vi "A 正面 处理函数.vi"(8 "error in (no error)":errorcluster caption="错误输入（无错误）", 10 "Image Name":string="I1", 11 "ParamsUI":T1 caption="参数界面" {"Exposure Values" scale=0.0..200000.0}) -> (0 "error out":errorcluster caption="错误输出", 3 "Image out":T3(plugin-control))   [LabVIEW 2015]
uses:
  <vilib>/userdefined/High Color/IMAQdx.ctl
  <resource>/objmgr/imaqdx.rc
  <vilib>/vision/driver/NI_Vision_Acquisition_Software.lvlib
panel:
  in  "Session Out":T2
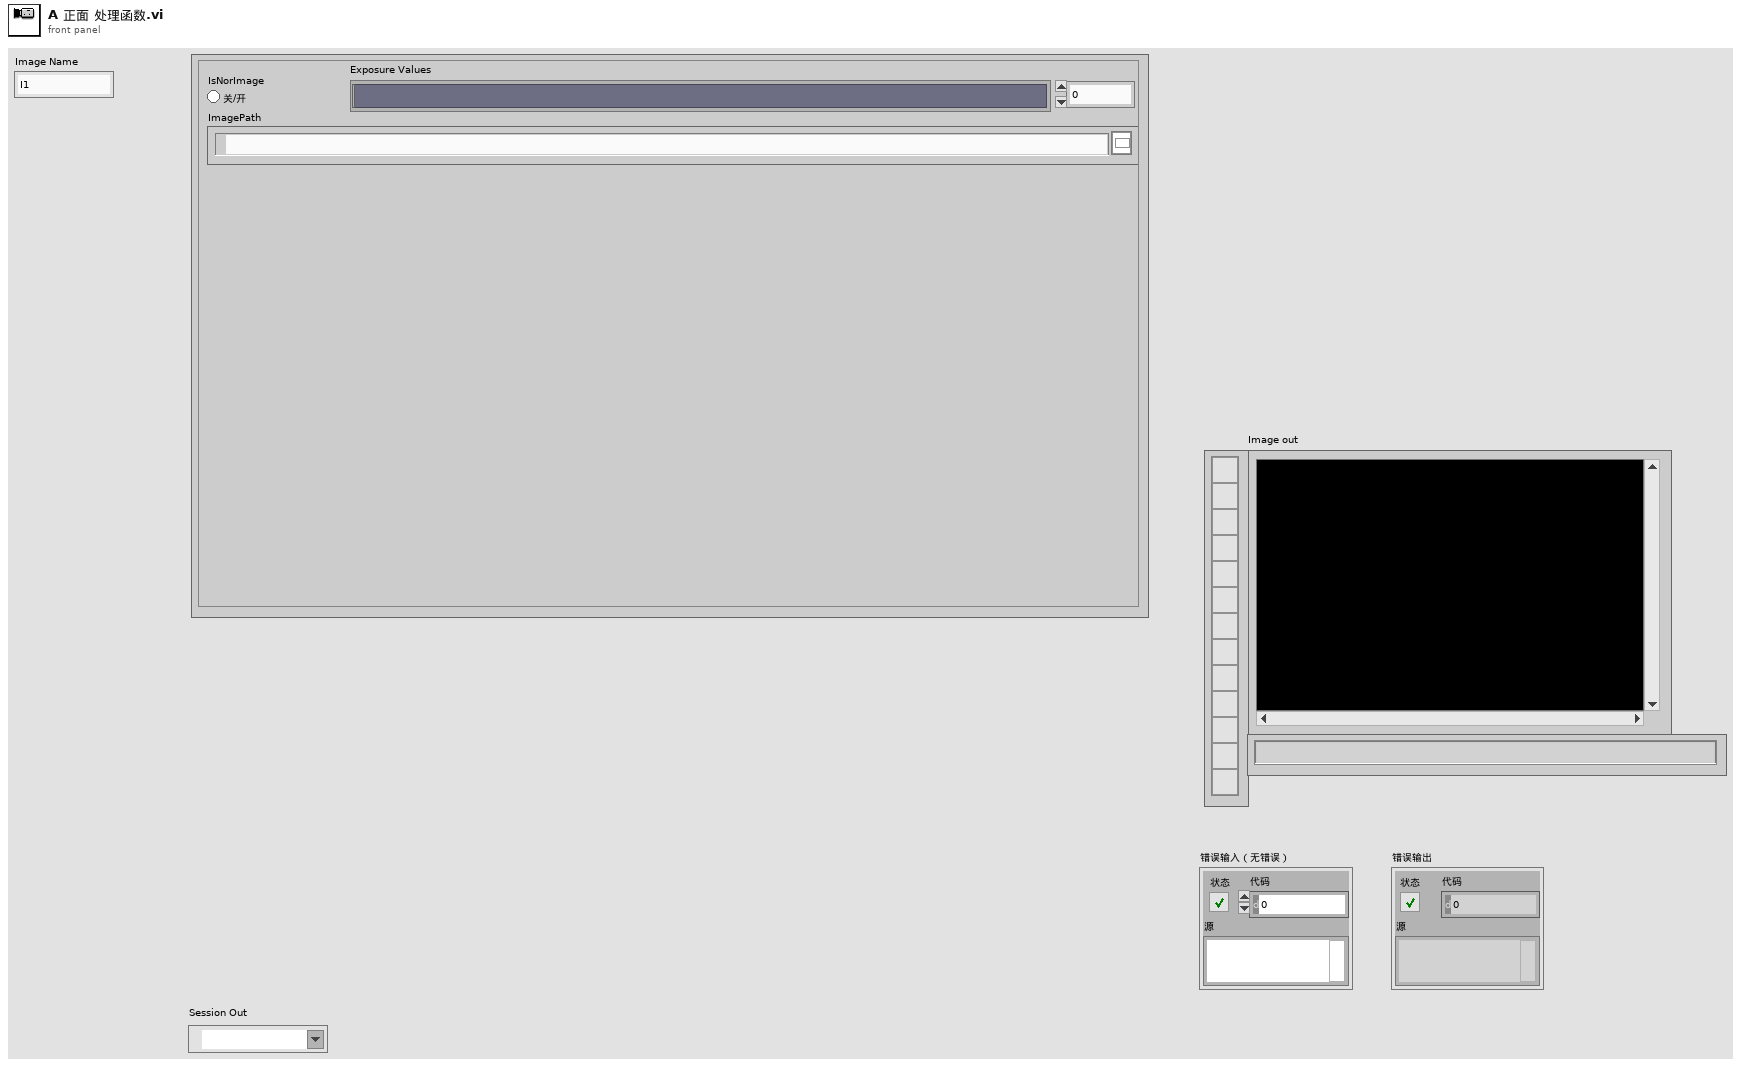
[diagram p1: front panel]
types:
  T1 = cluster{"IsNorImage":bool, "Exposure Values":u32, "ImagePath":path}
  T2 = typedef "IMAQdx.ctl" = refnum<k21>
  T3 = typedef "IMAQ Image.ctl" = refnum<image>
  T4 = typedef "Image Type" = u32
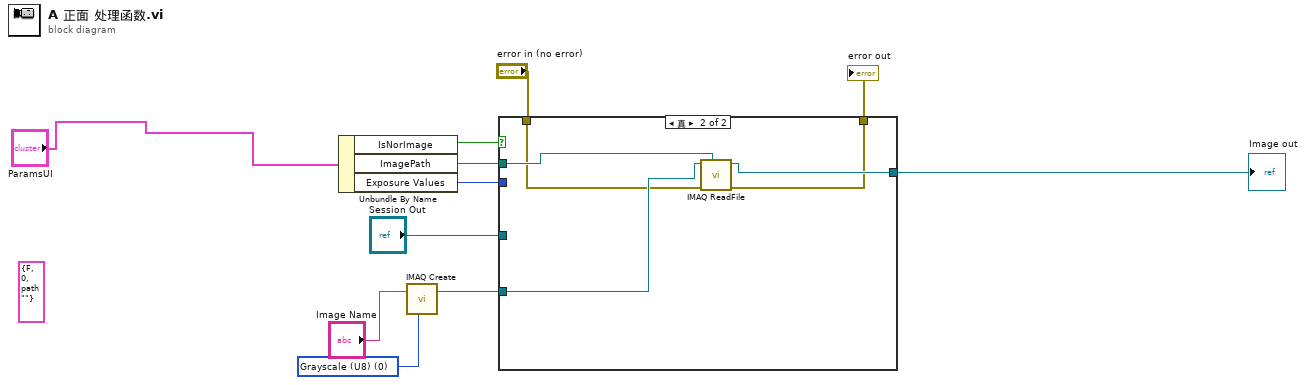
[diagram p0: block diagram]
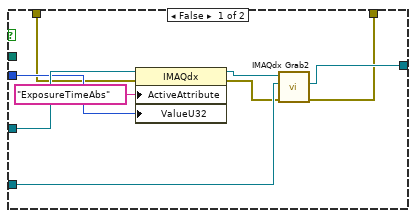
[diagram p2: hidden frame]
diagram:
  w1 = T4 0 items=["Grayscale (U8)", "Grayscale (I16)", "Grayscale (SGL)", "Complex (CSG)", "RGB (U32)", "HSL (U32)", "RGB (U64)", "Grayscale (U16)"] ("Image Type")
  (unwired) T1 {"IsNorImage"=FALSE, "Exposure Values"=0, "ImagePath"=path ""} ("ParamsUI")
  n1 = Unbundle By Name("ParamsUI") -> ("IsNorImage"=w11:bool, "ImagePath"=w10:path, "Exposure Values"=w8:u32)
  n2 = call "IMAQ Create"("Image Name"="Image Name", "Image Type"=w1) -> ("New Image"=w5:T3)  [unwired: 3 in, 1 out]
  n3 = case shown="真" w11 {
    tunnel: w10 -> [_ w25]
    tunnel: [w14 w24] -> w9
    tunnel: w8 -> [w18 _]
    tunnel: "Session Out" -> [w20 _]
    tunnel: w5 -> [w16 w23]
    tunnel: "error in (no error)" -> [w13 w22]
    tunnel: [w12 w21] -> w3
    frame False {
      n4 = property class="IMAQdx"(reference=w20, error in=w13, "ActiveAttribute"="ExposureTimeAbs", "ValueU32"=w18) -> (reference out=w17:T2, error out=w15:errorcluster)
      n5 = call <vilib>:"IMAQdx Grab2.vi"("error in"=w15, "Image In"=w16, "Session In"=w17) -> ("error out"=w12:errorcluster, "Image Out"=w14:T3)  [unwired: 5 in, 2 out]
    }
    frame True {
      n6 = call "IMAQ ReadFile"("File Path"=w25, "error in (no error)"=w22, "Image"=w23) -> ("error out"=w21:errorcluster, "Image Out"=w24:T3)  [unwired: 4 in, 3 out]
    }
  }
  "Image out" <- w9
  "error out" <- w3
